vi "CNR update TR radius.vi"(6 "TR update constants":cluster{"h1":dbl, "h2":dbl, "a1":dbl, "a2":dbl}={"h1"=0.0001, "h2"=0.99, "a1"=0.25, "a2"=3.5}, 7 "step":dbl[](array[numeric]), 8 "error in (no error)":errorcluster, 9 "L(0)-L(p_dl)":dbl, 10 "F(x)-F(x+p)":dbl, 11 "TR Radius":dbl) -> (0 "error out":errorcluster, 1 "quit?":bool, 2 "step OK?":bool, 3 "TR Radius out":dbl)   [LabVIEW 2020, in "NI_Gmath.lvlib"]
uses:
  <vilib>/gmath/NI_Gmath.lvlib
panel:
  # "basic trust region\n0<=h1 < h2 <1\n0<a1<1<a2"
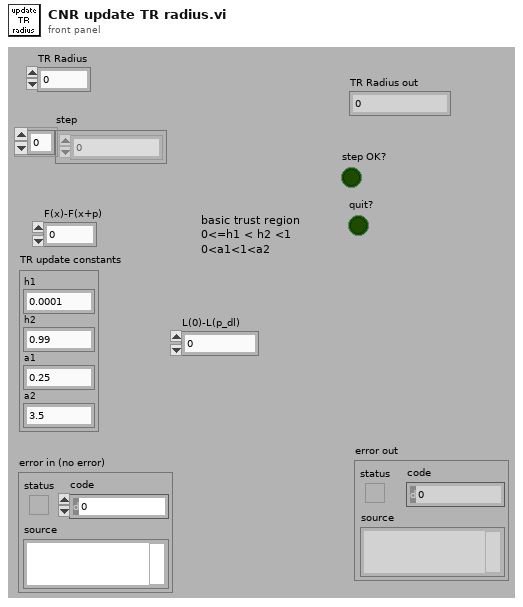
[diagram p1: front panel]
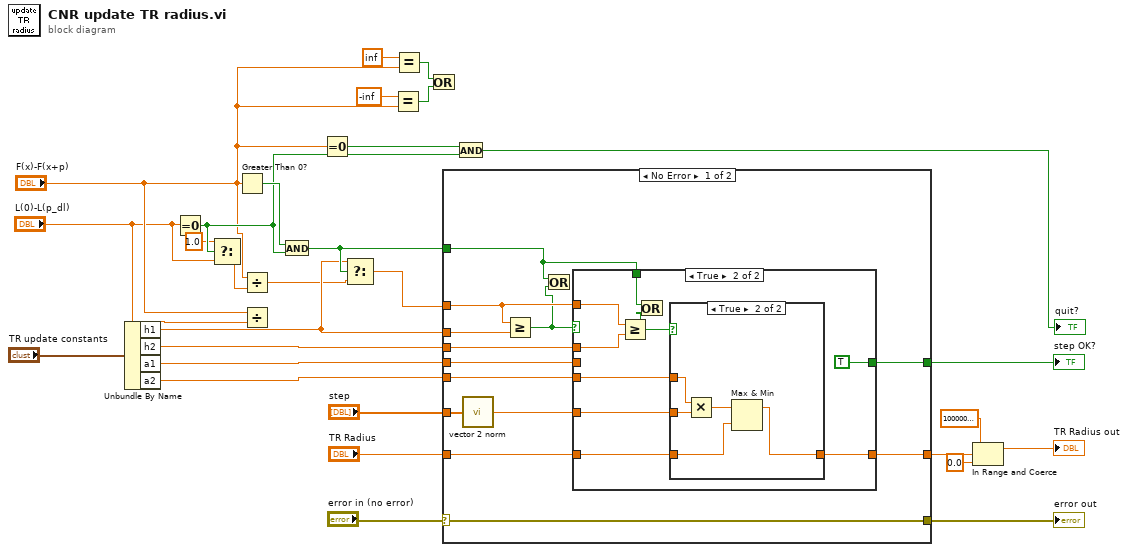
[diagram p0: block diagram]
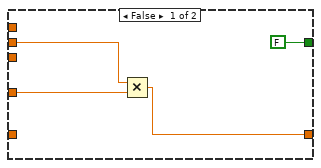
[diagram p2: hidden frame]
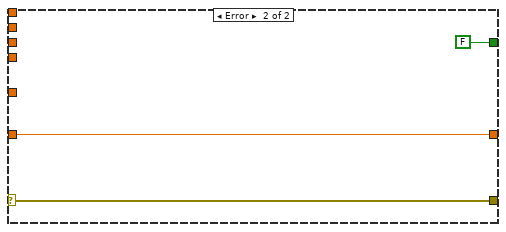
[diagram p4: hidden frame]
diagram:
  n1 = Unbundle By Name("TR update constants") -> ("h1"=w5:dbl, "h2"=w12:dbl, "a1"=w11:dbl, "a2"=w10:dbl)
  n2 = Equal To 0?(x="L(0)-L(p_dl)") -> (x = 0?=w9:bool)
  n3 = Select(t=1.0, s=w9, f="L(0)-L(p_dl)") -> (s? t:f=w7:dbl)
  n4 = Greater Than 0?(x="F(x)-F(x+p)") -> (x > 0?=w20:bool)
  n5 = Divide(x="F(x)-F(x+p)", y=w7) -> (x/y=w4:dbl)
  n6 = Divide(x="F(x)-F(x+p)", y="L(0)-L(p_dl)") -> ()  [unwired: 1 out]
  n7 = And(x=w20, y=w9) -> (x .and. y?=w6:bool)
  n8 = Equal To 0?(x="F(x)-F(x+p)") -> (x = 0?=w19:bool)
  n9 = Select(t=w5, s=w6, f=w4) -> (s? t:f=w1:dbl)
  n10 = Equal?(x=-inf, y="F(x)-F(x+p)") -> (x = y?=w14:bool)
  n11 = Equal?(x=inf, y="F(x)-F(x+p)") -> (x = y?=w15:bool)
  n12 = Or(x=w15, y=w14) -> ()  [unwired: 1 out]
  n13 = case shown="No Error" "error in (no error)" {
    selector: "error in (no error)" -> [w38 w64]
    tunnel: "step" -> [w37 _]
    tunnel: [w42 FALSE ("new step OK?")] -> w28
    tunnel: w1 -> [w41 _]
    tunnel: "TR Radius" -> [w40 w62]
    tunnel: [w39 w62] -> w21
    tunnel: [w38 w64] -> w25
    tunnel: w6 -> [w35 _]
    tunnel: w5 -> [w34 _]
    tunnel: w12 -> [w33 _]
    tunnel: w11 -> [w32 _]
    tunnel: w10 -> [w31 _]
    frame No Error {
      n14 = call <vilib>:"vector 2 norm.vi"("vector"=w37) -> ("vector2_norm"=w36:dbl)  [unwired: 14 in]
      n15 = Greater Or Equal?(x=w41, y=w34) -> (x >= y?=w30:bool)
      n16 = Or(x=w35, y=w30) -> ()  [unwired: 1 out]
      n17 = case shown="True" w30 {
        tunnel: [FALSE ("new step OK?") TRUE ("new step OK?")] -> w42
        tunnel: w41 -> [_ w55]
        tunnel: w33 -> [_ w54]
        tunnel: w31 -> [_ w53]
        tunnel: w32 -> [w45 _]
        tunnel: w36 -> [w44 w52]
        tunnel: w40 -> [_ w51]
        tunnel: [w43 w50] -> w39
        tunnel: w35 -> [_ w48]
        frame False {
          n18 = Multiply(x=w45, y=w44) -> (x*y=w43:dbl)
        }
        frame True {
          n19 = Greater Or Equal?(x=w55, y=w54) -> (x >= y?=w47:bool)
          n20 = Or(x=w48, y=w47) -> ()  [unwired: 1 out]
          n21 = case shown="True" w47 {
            tunnel: w53 -> [_ w60]
            tunnel: w52 -> [_ w61]
            tunnel: w51 -> [w56 w59]
            tunnel: [w56 w57] -> w50
            frame False {
            }
            frame True {
              n22 = Multiply(x=w60, y=w61) -> (x*y=w58:dbl)
              n23 = Max & Min(x=w58, y=w59) -> (max(x,y)=w57:dbl)  [unwired: 1 out]
            }
          }
        }
      }
    }
    frame Error {
    }
  }
  "step OK?" <- w28
  "error out" <- w25
  n24 = And(x=w19, y=w9) -> (x .and. y?=→"quit?":bool)
  n25 = In Range and Coerce(upper limit=1000000000000000.0, x=w21, lower limit=0.0) -> (coerced(x)=→"TR Radius out":dbl)  [unwired: 1 out]
